vi "decimateAllMatrix_singleAxis.vi"(10 "AllMatrix":dbl[](array[numeric]), 11 "NS":u8) -> (2 "ControlMatrices":T1, 4 "remaining_array":dbl[](array[numeric]))   [LabVIEW 2017]
uses:
  controls/ObserverMatrices.ctl
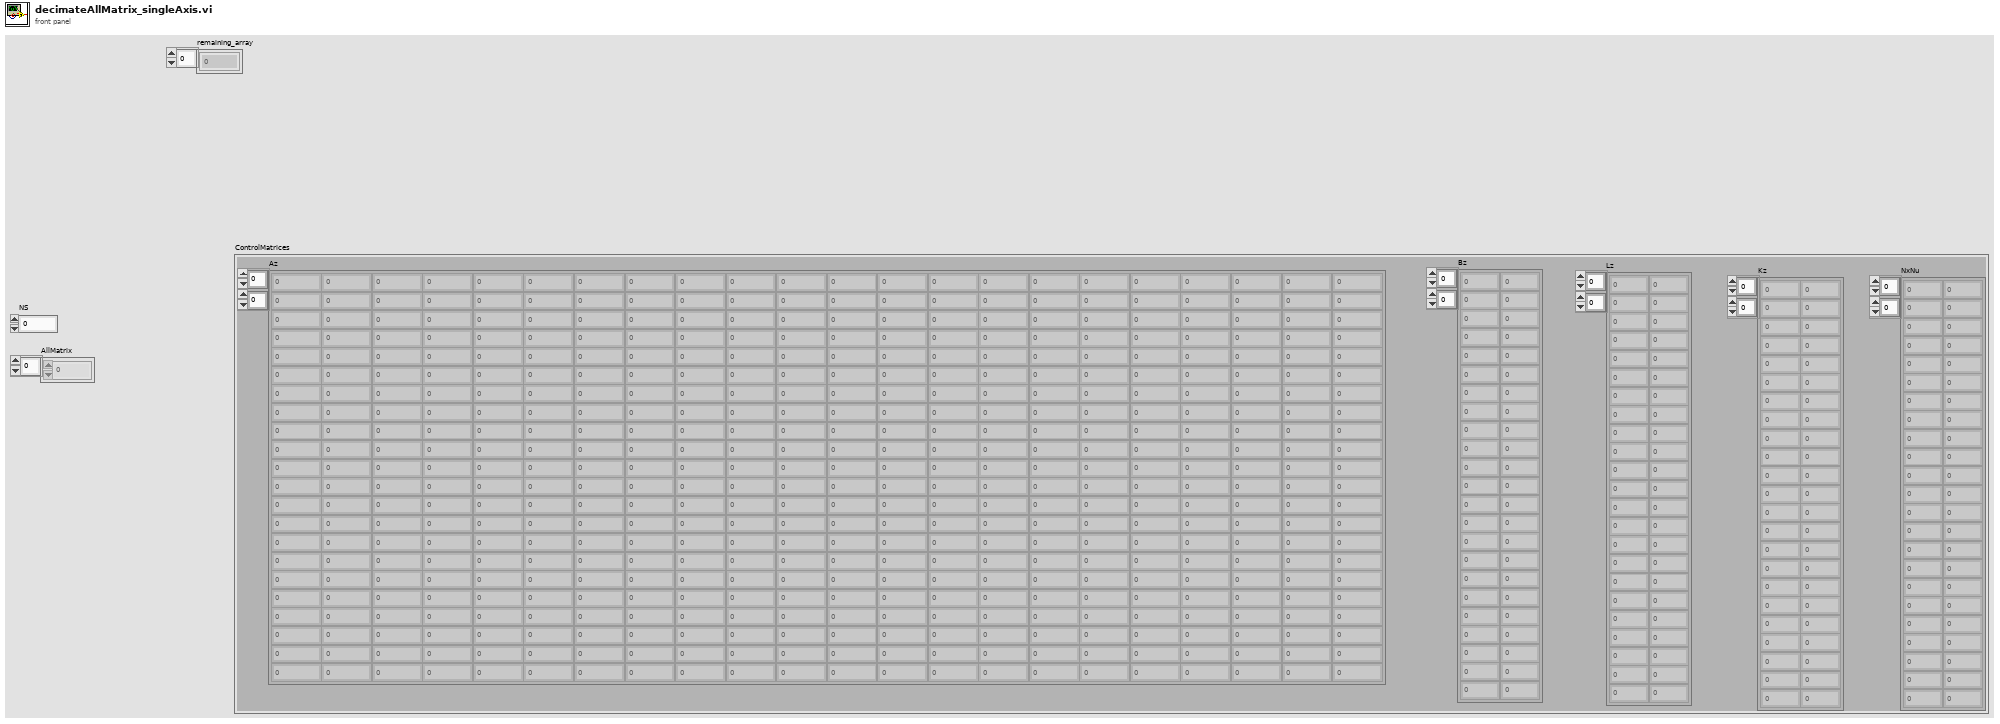
[diagram p1: front panel]
types:
  T1 = typedef "ObserverMatrices.ctl" = cluster{"Az":fxp<+/-,32,4>[][], "Bz":dbl[][], "Lz":dbl[][], "Kz":dbl[][], "NxNu":dbl[][]}
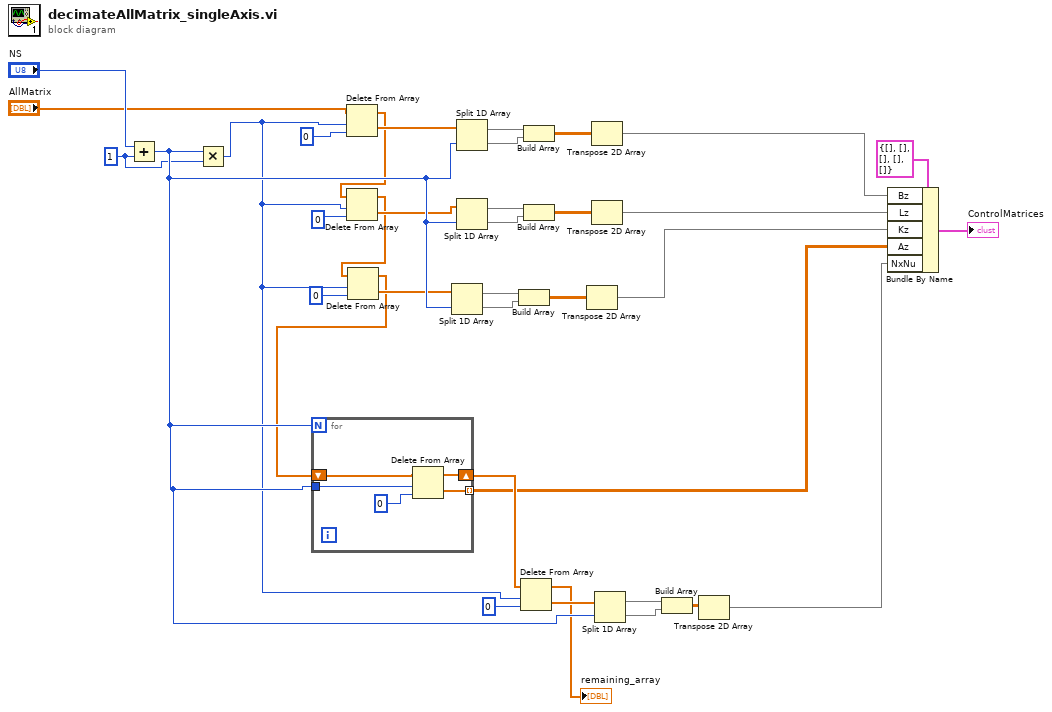
[diagram p0: block diagram]
diagram:
  w18 = u8 1 ("y")
  n1 = Add(x="NS", y=w18) -> (x+y=w37:u8)
  n2 = Multiply(x=w37, y=w18) -> (x*y=w20:u8)
  n3 = Delete From Array(array="AllMatrix", length=w20, index=0) -> (deleted portion=w23:dbl[], array with subset deleted=w10:dbl[])
  n4 = Delete From Array(array=w10, length=w20, index=0) -> (deleted portion=w28:dbl[], array with subset deleted=w12:dbl[])
  n5 = Delete From Array(array=w12, length=w20, index=0) -> (deleted portion=w32:dbl[], array with subset deleted=w19:dbl[])
  n6 = for {
    N: w37 -> [_]
    shift-right: [w38] -> w15
    shift-left: w19 -> [w41]
    tunnel: w37 -> [w40]
    tunnel: [w39] -> w4 mode=indexing
    n7 = Delete From Array(array=w41, length=w40, index=0) -> (deleted portion=w39:dbl[], array with subset deleted=w38:dbl[])
  }
  n8 = Split 1D Array(array=w32, index=w37) -> (first subarray=w29:dbl[], second subarray=w30:dbl[])
  n9 = Split 1D Array(array=w23, index=w37) -> (first subarray=w21:dbl[], second subarray=w22:dbl[])
  n10 = Split 1D Array(array=w28, index=w37) -> (first subarray=w25:dbl[], second subarray=w26:dbl[])
  n11 = Build Array(w29, w30) -> (w31:dbl[][])
  n12 = Delete From Array(array=w15, length=w20, index=0) -> (deleted portion=w36:dbl[], array with subset deleted=→"remaining_array":dbl[])
  n13 = Build Array(w21, w22) -> (w24:dbl[][])
  n14 = Build Array(w25, w26) -> (w27:dbl[][])
  n15 = Transpose 2D Array(2D array=w31) -> (transposed array=w6:dbl[][])
  n16 = Transpose 2D Array(2D array=w24) -> (transposed array=w8:dbl[][])
  n17 = Transpose 2D Array(2D array=w27) -> (transposed array=w7:dbl[][])
  n18 = Split 1D Array(array=w36, index=w37) -> (first subarray=w33:dbl[], second subarray=w34:dbl[])
  n19 = Build Array(w33, w34) -> (w35:dbl[][])
  n20 = Transpose 2D Array(2D array=w35) -> (transposed array=w3:dbl[][])
  n21 = Bundle By Name(cluster=T1 {"Az"=[], "Bz"=[], "Lz"=[], "Kz"=[], "NxNu"=[]} ("ControlMatrices 2"), "Bz"=w8, "Lz"=w7, "Kz"=w6, "Az"=w4, "NxNu"=w3) -> (→"ControlMatrices":T1)
